vi "PVcam_init_wrap.vi"(8 "error in (no error)":errorcluster) -> ()   [LabVIEW 2025]
uses:
  Windows/System32/pvcam64.dll
panel:
  out "error out":errorcluster
  out "return_bool":u16
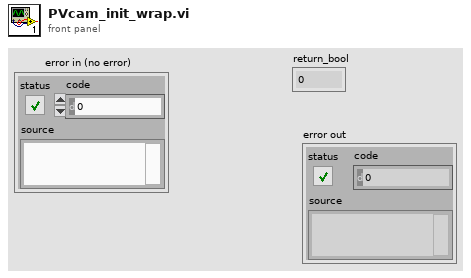
[diagram p1: front panel]
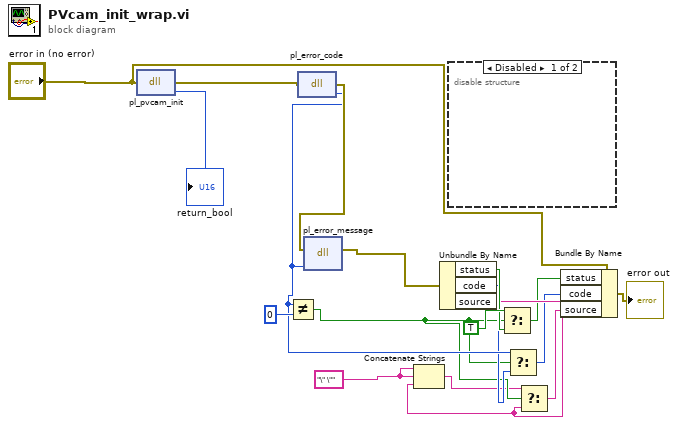
[diagram p0: block diagram]
diagram:
  w1 = "\" \"" ("string")
  n1 = dll-call lib="C:/Windows/System32/pvcam64.dll" fn="pl_pvcam_init"(error in="error in (no error)") -> (error out=w17:errorcluster, "return_bool"=→"return_bool":u16)  [unwired: 2 in, 1 out]
  n2 = dll-call lib="C:/Windows/System32/pvcam64.dll" fn="pl_error_code"(error in=w17) -> (error out=w16:errorcluster, "error code"=w11:u16)  [unwired: 2 in, 1 out]
  n3 = Not Equal?(x=w11, y=u16 0) -> (x != y?=w9:bool)
  n4 = dll-call lib="C:/Windows/System32/pvcam64.dll" fn="pl_error_message"(error in=w16, "error_code"=w11) -> (error out=w15:errorcluster)  [unwired: 4 in, 1 out]
  n5 = Unbundle By Name(w15) -> ("status"=w12:bool, "code"=w10:i32, "source"=w7:string)
  n6 = Concatenate Strings(w1, w1, w7) -> (w8:string)
  n7 = disable-structure shown="Disabled" {
    frame Disabled {
    }
    frame Enabled {
    }
  }
  n8 = Select(t=TRUE, s=w9, f=w12) -> (s? t:f=w3:bool)
  n9 = Select(t=w11, s=w9, f=w10) -> (s? t:f=w4:i32)
  n10 = Select(t=w8, s=w9, f=w7) -> (s? t:f=w5:string)
  n11 = Bundle By Name(cluster="error in (no error)", "status"=w3, "code"=w4, "source"=w5) -> (→"error out":errorcluster)
